vi "View.vi"(8 "error in (no error)":errorcluster, 11 "Recipe View in":refnum<class "Recipe View.lvclass">) -> (0 "error out":errorcluster, 3 "Recipe View out":refnum<class "Recipe View.lvclass">)   [LabVIEW 2022 SP3, in "Recipe View.lvclass"]
uses:
  Recipe View.lvclass
  C:/XY Stage/iView/base view/base view.lvclass
  Laser/Laser State Data/Laser State.ctl
  Recipe State Data/Recipe State Data.lvclass/Recipe State Data.ctl
  Recipe State Data/Write Recipe Data Save Location.vi
  Recipe State Data/Read Recipe Data Save Location.vi
  Accessors/Read Recipe API.lvclass.vi
  iView/base view/Accessors/Read Events.vi
  Accessors/Read 2-Axis Stage Status.lvclass.vi
  Accessors/Read Camera Async Coms.lvclass.vi
  Accessors/Read Get Daq Status.lvclass.vi
  Accessors/Read Get Laser Status.lvclass.vi
  Accessors/Read XY stage VIEW.vi
  Accessors/Read Laser VIEW.vi
  Accessors/Read Camera VIEW.vi
  Accessors/Read DAQ VIEW.vi
  iView/base view/base view.lvclass
  Recipe API/Recipe API.lvclass
  XY Stage/Interfaces/Async Coms/Async Coms.lvclass
  Camera/Camera Async Coms/Camera Async Coms.lvclass
  IO Monitor/Get Daq Status/Get Daq Status.lvclass
  Laser/Get Laser Status/Get Laser Status.lvclass
  Recipe View.lvclass/Recipe View.ctl
  Recipe State Data/Recipe State Data.lvclass
  Laser/Laser State Data/Laser State Data.lvclass
panel:
  in  "Views":enum32{"XY Stage", "Laser", "Camera", "DAQ"}(radio)
  out "XY Position Graph":cluster{"X":dbl, "Y":dbl}[](graph)
  out "XY Graph":T1(graph)
  out "Current Laser Power%":dbl
  out "Stage Homed":bool
  out "Laser Temp(c)":dbl
  out "Laser State":T2
  out "DAQ Acquiring":bool
  out "Camera Saving":bool
  in  "Recipe Data Output":path=path "C:/Data/Recipe output"
  in  "Recipe File":path=path "C:/Data/Recipes"
  in  "Stop Recipe":bool
  in  "Start Recipe":bool
  out "Recipe Iterations":dbl
  out "Desired Recipe Iterations":dbl
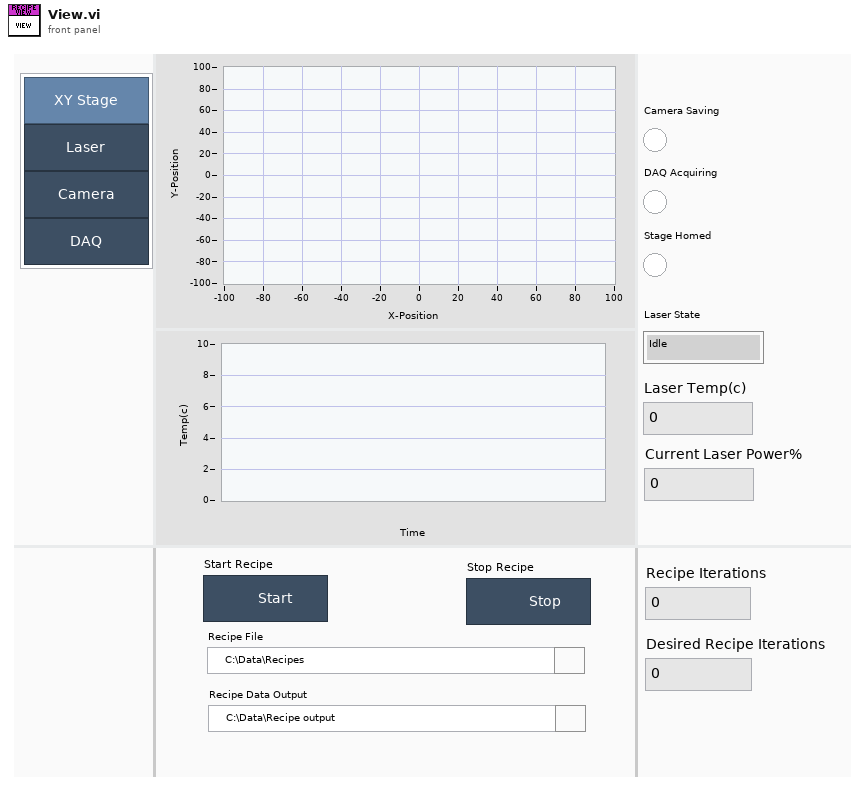
[diagram p1: front panel]
types:
  T1 = cluster{"AI Channel Data":cluster{"Time Stamp":timestamp, "AI":dbl}[]}[]
  T2 = typedef "Laser State Data.lvclass/Laser State.ctl" = enum16{"Idle", "Warming", "Ready", "Firing"}
  T3 = typedef "base view.lvclass/Events.ctl" = cluster{"Open":refnum<user-event>, "Close":refnum<user-event>, "Hide":refnum<user-event>}
  T4 = cluster{"Event Registration Refnum":refnum<event-registration>, "Event Registration Refnum":refnum<event-registration>}
  T5 = cluster{"Event Registration Refnum":refnum<event-registration>, "Recipe Process":refnum<event-registration>, "Recipe State":refnum<event-registration>, "Event Registration Refnum":refnum<event-registration>, "Event Registration Refnum":refnum<event-registration>, "Event Registration Refnum":refnum<event-registration>, "Event Registration Refnum":refnum<event-registration>, "Daq events":refnum<event-registration>, "Process State":refnum<event-registration>, "Laser State":refnum<event-registration>}
  T6 = enum8{"Enabled", "Disabled", "Disabled and Grayed Out"}
  T7 = cluster{"Current Position X":dbl, "Current Position Y":dbl}[]
  T8 = typedef "AI Daq Data.lvlib/AIDAQ Data.ctl" = cluster{"Time Stamp":timestamp, "AI":dbl}
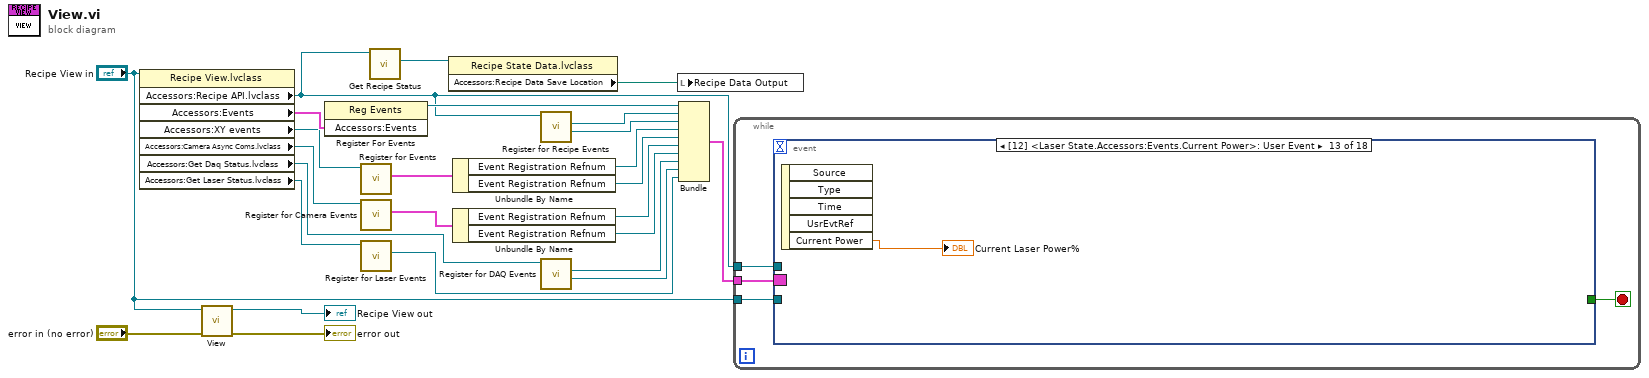
[diagram p0: block diagram]
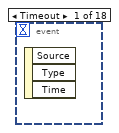
[diagram p2: hidden frame]
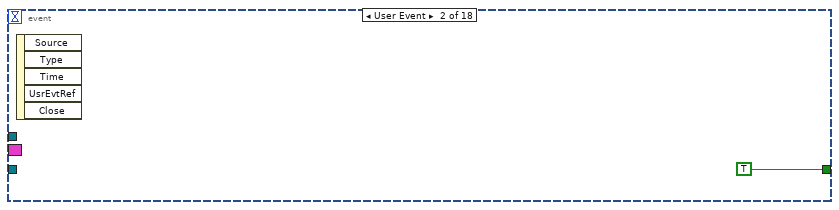
[diagram p3: hidden frame]
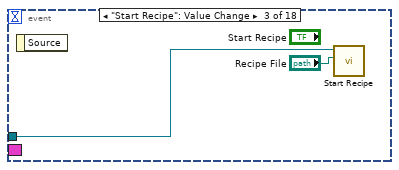
[diagram p4: hidden frame]
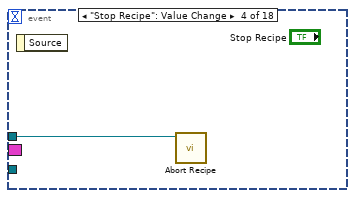
[diagram p5: hidden frame]
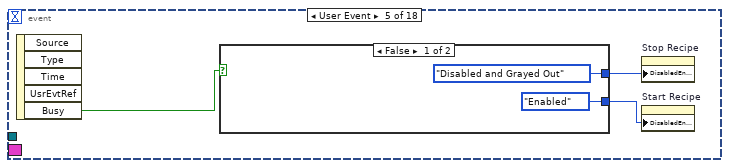
[diagram p6: hidden frame]
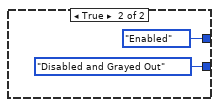
[diagram p7: hidden frame]
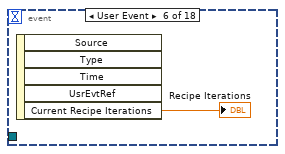
[diagram p8: hidden frame]
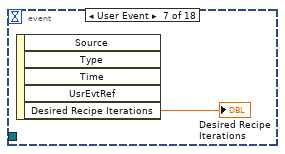
[diagram p9: hidden frame]
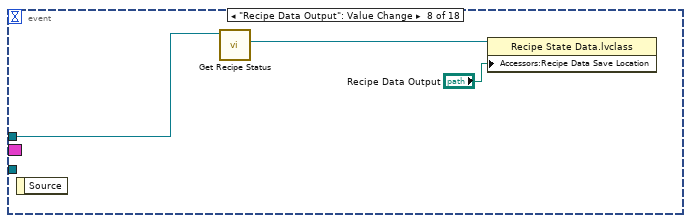
[diagram p10: hidden frame]
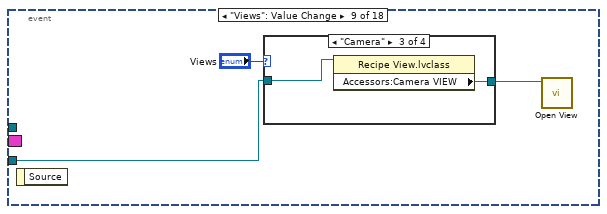
[diagram p11: hidden frame]
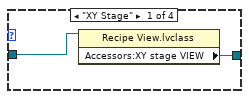
[diagram p12: hidden frame]
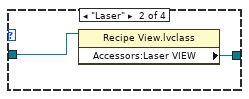
[diagram p13: hidden frame]
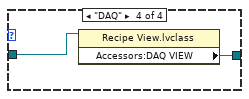
[diagram p14: hidden frame]
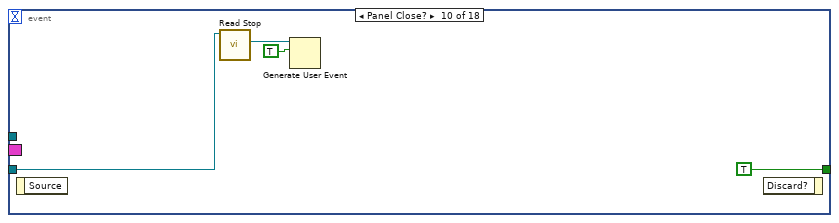
[diagram p15: hidden frame]
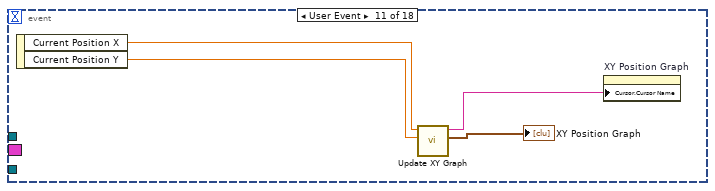
[diagram p16: hidden frame]
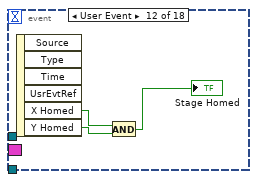
[diagram p17: hidden frame]
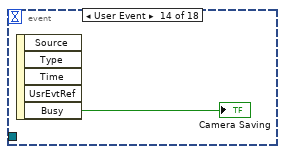
[diagram p18: hidden frame]
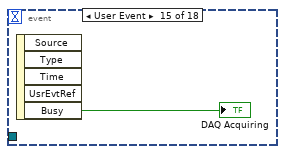
[diagram p19: hidden frame]
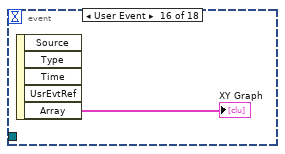
[diagram p20: hidden frame]
diagram:
  n1 = property class="Recipe View.lvclass"(reference="Recipe View in") -> ("Accessors:Recipe API.lvclass"=w16:refnum<class "Recipe API.lvclass">, "Accessors:Events"=w22:T3, "Accessors:XY events"=w13:refnum<class "Async Coms.lvclass">, "Accessors:Camera Async Coms.lvclass"=w9:refnum<class "Camera Async Coms.lvclass">, "Accessors:Get Daq Status.lvclass"=w5:refnum<class "Get Daq Status.lvclass">, "Accessors:Get Laser Status.lvclass"=w2:refnum<class "Get Laser Status.lvclass">)  [unwired: 1 in, 2 out]
  n2 = call-parent "View.vi"("error in (no error)"="error in (no error)", "base view in"="Recipe View in") -> ("error out"=→"error out":errorcluster, "base view out"=→"Recipe View out":refnum<class "Recipe View.lvclass">)  [unwired: 8 in]
  n3 = register-events(w22) -> (reference out=w21:refnum<event-registration>)  [unwired: 2 in, 1 out]
  n4 = call-dynamic "Register for Events.vi"("Async Coms in"=w13) -> ("Event Refnums"=w12:T4)  [unwired: 8 in, 2 out]
  n5 = call-dynamic "Register for Camera Events.vi"("Camera Async Coms in"=w9) -> ("output cluster"=w8:T4)  [unwired: 8 in, 2 out]
  n6 = call-dynamic "Register for Laser Events.vi"("Get Laser Status in"=w2) -> ("Laser State"=w1:refnum<event-registration>)  [unwired: 7 in, 3 out]
  n7 = call-dynamic "Get Recipe Status.vi"("Recipe Status in"=w16) -> ("Recipe State Data"=w17:refnum<data-value>)  [unwired: 8 in, 2 out]
  n8 = property class="Recipe State Data.lvclass"(reference=w17) -> ("Accessors:Recipe Data Save Location"=w15:path)  [unwired: 1 in, 2 out]
  n9 = Unbundle By Name(w12) -> ("Event Registration Refnum"=w11:refnum<event-registration>, "Event Registration Refnum"=w10:refnum<event-registration>)
  n10 = Unbundle By Name(w8) -> ("Event Registration Refnum"=w7:refnum<event-registration>, "Event Registration Refnum"=w6:refnum<event-registration>)
  n11 = call-dynamic "Register for Recipe Events.vi"("Recipe Status in"=w16) -> ("Recipe State"=w18:refnum<event-registration>, "Recipe Process"=w19:refnum<event-registration>)  [unwired: 7 in, 2 out]
  n12 = call-dynamic "Register for DAQ Events.vi"("Get Daq Status in"=w5) -> ("Process State"=w3:refnum<event-registration>, "Daq events"=w4:refnum<event-registration>)  [unwired: 7 in, 2 out]
  n13 = local write "Recipe Data Output"(w15) -> ()
  n14 = Bundle("Event Registration Refnum"=w21, "Recipe Process"=w19, "Recipe State"=w18, "Event Registration Refnum"=w11, "Event Registration Refnum"=w10, "Event Registration Refnum"=w7, "Event Registration Refnum"=w6, "Daq events"=w4, "Process State"=w3, "Laser State"=w1) -> (w20:T5)  [unwired: 1 in]
  n15 = while {
    tunnel: w16 -> [w29]
    tunnel: w20 -> [w28]
    tunnel: "Recipe View in" -> [w26]
    stop <- w27 stop-if-true
    n16 = event shown="[12] <Laser State.Accessors:Events.Current Power>: User Event" {
      selector: w28 -> [_ _ _ _ _ _ _ _ _ _ _ _ _ _ _ _ _ _]
      dyn-events: _ -> [_ _ _ _ _ _ _ _ _ _ _ _ _ _ _ _ _ _]
      timeout: _ -> [_ _ _ _ _ _ _ _ _ _ _ _ _ _ _ _ _ _]
      tunnel: w29 -> [_ _ w32 w33 _ _ _ w45 _ _ _ _ _ _ _ _ _ _]
      tunnel: [_ TRUE _ _ _ _ _ _ _ TRUE _ _ _ _ _ _ _ _] -> w27
      tunnel: w26 -> [_ _ _ _ _ _ _ _ w48 w59 _ _ _ _ _ _ _ _]
      event Timeout {
        n17 = event-data() -> ()  [unwired: 1 in, 3 out]
      }
      event User Event {
        n18 = event-data() -> ()  [unwired: 1 in, 5 out]
      }
      event "Start Recipe": Value Change {
        n19 = event-data() -> ()  [unwired: 1 in, 1 out]
        n20 = call-dynamic "Start Recipe.vi"("Recipe File"="Recipe File", "Recipe in"=w32) -> ()  [unwired: 8 in, 2 out]
      }
      event "Stop Recipe": Value Change {
        n21 = event-data() -> ()  [unwired: 1 in, 1 out]
        n22 = call-dynamic "Abort Recipe.vi"("Recipe in"=w33) -> ()  [unwired: 9 in, 2 out]
      }
      event User Event {
        n23 = event-data() -> ("Busy"=w36:bool)  [unwired: 1 in, 4 out]
        n24 = case shown="False" w36 {
          tunnel: [T6."Enabled" ("Disabled") T6."Disabled and Grayed Out" ("Disabled")] -> w35
          tunnel: [T6."Disabled and Grayed Out" ("Disabled") T6."Enabled" ("Disabled")] -> w34
          frame False {
          }
          frame True {
          }
        }
        n25 = property on="Stop Recipe" class="Bool"("DisabledEnum"=w34) -> ()  [unwired: 2 in, 2 out]
        n26 = property on="Start Recipe" class="Bool"("DisabledEnum"=w35) -> ()  [unwired: 2 in, 2 out]
      }
      event User Event {
        n27 = event-data() -> ("Current Recipe Iterations"=→"Recipe Iterations":dbl)  [unwired: 1 in, 4 out]
      }
      event User Event {
        n28 = event-data() -> ("Desired Recipe Iterations"=→"Desired Recipe Iterations":dbl)  [unwired: 1 in, 4 out]
      }
      event "Recipe Data Output": Value Change {
        n29 = event-data() -> ()  [unwired: 1 in, 1 out]
        n30 = call-dynamic "Get Recipe Status.vi"("Recipe Status in"=w45) -> ("Recipe State Data"=w44:refnum<data-value>)  [unwired: 8 in, 2 out]
        n31 = property class="Recipe State Data.lvclass"(reference=w44, "Accessors:Recipe Data Save Location"="Recipe Data Output") -> ()  [unwired: 1 in, 2 out]
      }
      event "Views": Value Change {
        n32 = event-data() -> ()  [unwired: 1 in, 1 out]
        n33 = case shown="\"Camera\"" "Views" {
          tunnel: w48 -> [w50 w52 w54 w56]
          tunnel: [w49 w51 w53 w55] -> w46
          frame "XY Stage" {
            n34 = property class="Recipe View.lvclass"(reference=w50) -> ("Accessors:XY stage VIEW"=w49:refnum<class "base view.lvclass">)  [unwired: 1 in, 2 out]
          }
          frame "Laser" {
            n35 = property class="Recipe View.lvclass"(reference=w52) -> ("Accessors:Laser VIEW"=w51:refnum<class "base view.lvclass">)  [unwired: 1 in, 2 out]
          }
          frame "Camera" {
            n36 = property class="Recipe View.lvclass"(reference=w54) -> ("Accessors:Camera VIEW"=w53:refnum<class "base view.lvclass">)  [unwired: 1 in, 2 out]
          }
          frame "DAQ" {
            n37 = property class="Recipe View.lvclass"(reference=w56) -> ("Accessors:DAQ VIEW"=w55:refnum<class "base view.lvclass">)  [unwired: 1 in, 2 out]
          }
        }
        n38 = call-dynamic "Open View.vi"("base view in"=w46) -> ()  [unwired: 9 in, 2 out]
      }
      event Panel Close? {
        n39 = event-data() -> ()  [unwired: 1 in, 1 out]
        n40 = call "Read Stop.vi"("In"=w59) -> ("Stop"=w58:refnum<user-event>)  [unwired: 8 in, 2 out]
        n41 = Generate User Event(user event=w58, event data cluster=TRUE) -> ()  [unwired: 2 in, 2 out]
        n42 = event-data() -> ()  [unwired: 2 in, 1 out]
      }
      event User Event {
        n43 = event-data() -> ("Current Position X"=w64:dbl, "Current Position Y"=w63:dbl)  [unwired: 1 in]
        n44 = call "Update XY Graph.vi"("Current Position Y"=w63, "Current Position X"=w64) -> ("Array"=→"XY Position Graph":T7, "String"=w61:string)  [unwired: 7 in, 1 out]
        n45 = property on="XY Position Graph" class="XYGraph (strict)"("Cursor.Cursor Name"=w61) -> ()  [unwired: 2 in, 2 out]
      }
      event User Event {
        n46 = event-data() -> ("X Homed"=w67:bool, "Y Homed"=w66:bool)  [unwired: 1 in, 4 out]
        n47 = And(x=w67, y=w66) -> (x .and. y?=→"Stage Homed":bool)
      }
      event User Event {
        n48 = event-data() -> ("Current Power"=→"Current Laser Power%":dbl)  [unwired: 1 in, 4 out]
      }
      event User Event {
        n49 = event-data() -> ("Busy"=→"Camera Saving":bool)  [unwired: 1 in, 4 out]
      }
      event User Event {
        n50 = event-data() -> ("Busy"=→"DAQ Acquiring":bool)  [unwired: 1 in, 4 out]
      }
      event User Event {
        n51 = event-data() -> ("Array"=→"XY Graph":cluster{"AI Channel Data":T8[]}[])  [unwired: 1 in, 4 out]
      }
      event User Event {
        n52 = event-data() -> ("Laser State"=→"Laser State":T2)  [unwired: 1 in, 4 out]
      }
      event User Event {
        n53 = event-data() -> ("Temp"=→"Laser Temp(c)":dbl)  [unwired: 1 in, 4 out]
      }
    }
  }
